vi "createFileStruc.vi"(8 "i_iter":i32, 9 "i_delay":i32, 11 "meas_path":path) -> (1 "AVG file":path, 2 "RAW file":path)   [LabVIEW 2020]
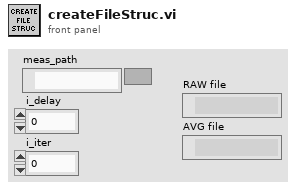
[diagram p1: front panel]
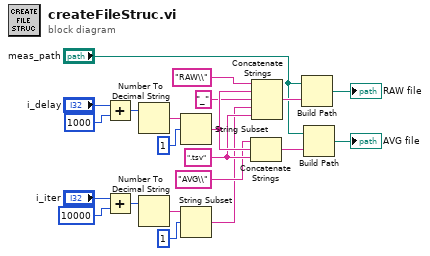
[diagram p0: block diagram]
diagram:
  w20 = ".tsv" ("string")
  n1 = Add(x="i_delay", y=1000) -> (x+y=w12:i32)
  n2 = Add(x="i_iter", y=10000) -> (x+y=w7:i32)
  n3 = Number To Decimal String(number=w12) -> (decimal integer string=w13:string)  [unwired: 1 in]
  n4 = Number To Decimal String(number=w7) -> (decimal integer string=w8:string)  [unwired: 1 in]
  n5 = String Subset(string=w13, offset (0)=1) -> (substring=w21:string)  [unwired: 1 in]
  n6 = String Subset(string=w8, offset (0)=1) -> (substring=w4:string)  [unwired: 1 in]
  n7 = Concatenate Strings("AVG\\" ("string"), w21, w20) -> (w18:string)
  n8 = Concatenate Strings("RAW\\" ("string"), w21, "_" ("string"), w4, w20) -> (w16:string)
  n9 = Build Path(base path="meas_path", name or relative path=w16) -> (appended path=→"RAW file":path)
  n10 = Build Path(base path="meas_path", name or relative path=w18) -> (appended path=→"AVG file":path)
